vi "PID Configuration.vi"(8 "error in (no error)":errorcluster, 10 "Parameters In":variant, 11 "Subpanel Queue In":refnum<queue>) -> (0 "error out":errorcluster, 2 "Parameters Out":variant)   [LabVIEW 2018]
doc: "Configuration control for the 'Set PID Configuration' step."
uses:
  controls/Control Configuration.ctl
panel:
  in  "Channel 0 Configuration":T1={"PID Gains"={"proportional gain (Kc)"=0.0, "integral gain (Kc*Ts/Ti)"=0.0, "derivative gain (Kc*Td/Ts)"=0.0}, "Output Range"={"output high"=10.0, "output low"=-10.0}}
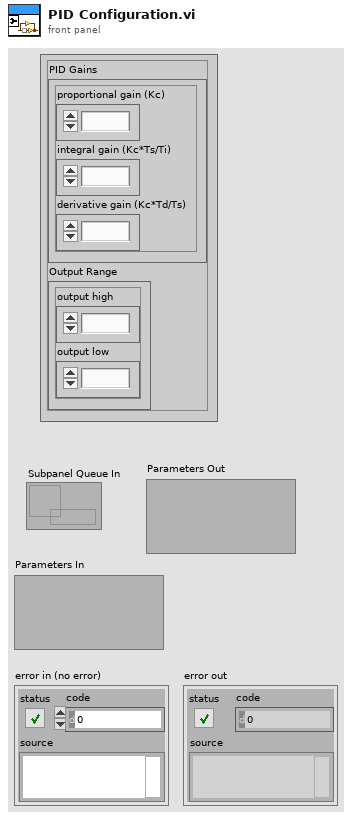
[diagram p1: front panel]
types:
  T1 = typedef "Control Configuration.ctl" = cluster{"PID Gains":cluster{"proportional gain (Kc)":fxp<+/-,16,8>, "integral gain (Kc*Ts/Ti)":fxp<+/-,16,8>, "derivative gain (Kc*Td/Ts)":fxp<+/-,16,8>}, "Output Range":cluster{"output high":fxp<+/-,16,5>, "output low":fxp<+/-,16,5>}}
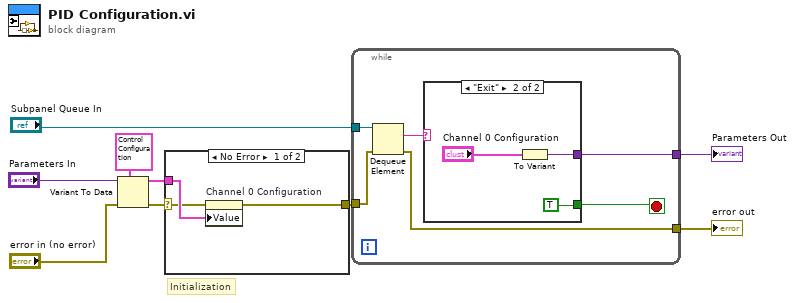
[diagram p0: block diagram]
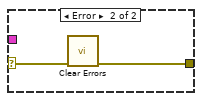
[diagram p2: hidden frame]
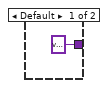
[diagram p3: hidden frame]
diagram:
  # "Initialization"
  n1 = Variant To Data(error in="error in (no error)", type=T1 {"PID Gains"={"proportional gain (Kc)"=0.0, "integral gain (Kc*Ts/Ti)"=0.0, "derivative gain (Kc*Td/Ts)"=0.0}, "Output Range"={"output high"=10.0, "output low"=-10.0}} ("Channel 0 Configuration"), Variant="Parameters In") -> (data=w7:T1, error out=w5:errorcluster)
  n2 = case shown="No Error" w5 {
    selector: w5 -> [w11 w14]
    tunnel: w7 -> [w12 _]
    tunnel: [w10 w13] -> w6
    frame No Error {
      n3 = property on="Channel 0 Configuration" class="Clust (strict)"(error in=w11, "Value"=w12) -> (error out=w10:errorcluster)  [unwired: 1 in, 1 out]
    }
    frame Error {
      n4 = call <vilib>:"Clear Errors.vi"("error in (no error)"=w14) -> ("error out"=w13:errorcluster)  [unwired: 5 in, 1 out]
    }
  }
  n5 = while {
    tunnel: "Subpanel Queue In" -> [w20]
    tunnel: w6 -> [w19]
    tunnel: [w17] -> w4
    tunnel: [w15] -> w1
    stop <- w16 stop-if-true
    n6 = Dequeue Element(queue=w20, error in (no error)=w19) -> (element=w18:string, error out=w15:errorcluster)  [unwired: 1 in, 2 out]
    n7 = case shown="\"Exit\"" w18 {
      tunnel: [variant ("Variant") w24] -> w17
      tunnel: [_ TRUE] -> w16
      frame Default {
      }
      frame "Exit" {
        n8 = To Variant(anything="Channel 0 Configuration") -> (Variant=w24:variant)
      }
    }
  }
  "Parameters Out" <- w4
  "error out" <- w1
